vi "New Data Logging Specification (Text).vi"(5 "Decimal Places (3)":u32=3, 6 "Header Text (\"\")":string, 7 "Delimiter (Tab)":T2, 8 "error in (no error)":errorcluster, 9 "Channel Paths":T1[](array[typedef]), 10 "File Conflict Operation":T3, 11 "Base Log File Path":path) -> (0 "error out":errorcluster, 3 "Data Logging Specification Ref out":T4)   [LabVIEW 2020, in "NI_VS Data Logging API.lvlib"]
doc: "Creates a new data logging specification, which defines the channels to log and the type and base path for log files. You can log data to TDMS or text (.txt) files. You must manually select the polymorphic instance to use."
uses:
  <vilib>/NI VeriStand/Execution/DataLogging/NI_VS Data Logging API.lvlib
  <vilib>/NI VeriStand/Execution/DataLogging/DataLoggingSpecification Ref.ctl
  NationalInstruments.VeriStand.ClientAPI
  <vilib>/NI VeriStand/Execution/DataLogging/File Conflict Operation.ctl
  <vilib>/NI VeriStand/Execution/DataLogging/Delimiter.ctl
  <vilib>/NI VeriStand/Execution/DataLogging/Text Channel.ctl
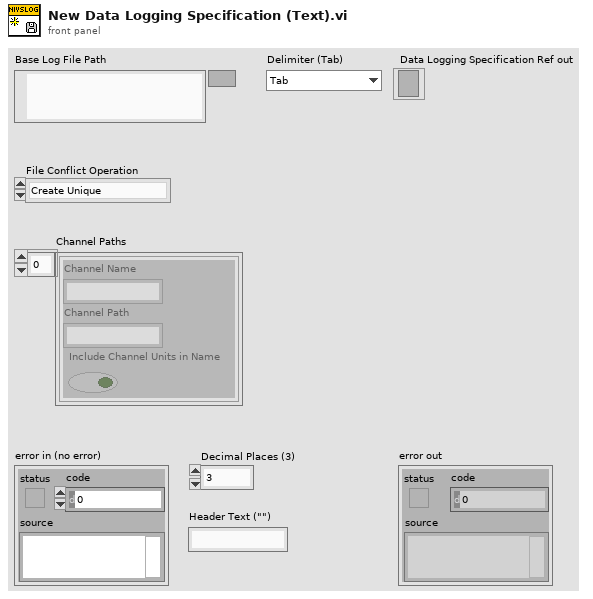
[diagram p1: front panel]
types:
  T1 = typedef "NI_VS Data Logging API.lvlib/Text Channel.ctl" = cluster{"Channel Name":string, "Channel Path":string, "Include Channel Units in Name":bool}
  T2 = typedef "NI_VS Data Logging API.lvlib/Delimiter.ctl" = enum16{"Tab", "Comma"}
  T3 = typedef "NI_VS Data Logging API.lvlib/File Conflict Operation.ctl" = enum16{"Create Unique", "Append to Existing", "Overwrite"}
  T4 = typedef "NI_VS Data Logging API.lvlib/DataLoggingSpecification Ref.ctl" = refnum<k24>
  T5 = typedef "NI_VS Data Logging API.lvlib/TextLogFile Ref.ctl" = refnum<k24>
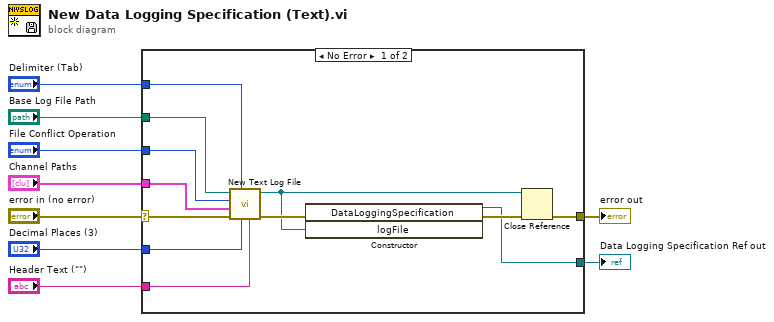
[diagram p0: block diagram]
diagram:
  n1 = case shown="No Error" "error in (no error)" {
    selector: "error in (no error)" -> [w16 w22]
    tunnel: [w18 _] -> w8
    tunnel: [w17 w22] -> w7
    tunnel: "File Conflict Operation" -> [w15 _]
    tunnel: "Base Log File Path" -> [w14 _]
    tunnel: "Delimiter (Tab)" -> [w13 _]
    tunnel: "Channel Paths" -> [w12 _]
    tunnel: "Decimal Places (3)" -> [w11 _]
    tunnel: "Header Text (\"\")" -> [w10 _]
    frame No Error {
      n2 = call <vilib>:"New Text Log File.vi"("Header Text (\"\")"=w10, "Decimal Places (3)"=w11, "Delimiter (Tab)"=w13, "error in (no error)"=w16, "Channel Paths"=w12, "File Conflict Operation"=w15, "Log File Path"=w14) -> ("error out"=w21:errorcluster, "TextLogFile Ref"=w19:T5)  [unwired: 3 in]
      n3 = constructor class="DataLoggingSpecification"(error in=w21, "logFile"=w19) -> (reference out=w18:refnum<k24>, error out=w20:errorcluster)  [unwired: 2 in, 2 out]
      n4 = Close Reference(reference=w19, error in (no error)=w20) -> (error out=w17:errorcluster)
    }
    frame Error {
    }
  }
  "error out" <- w7
  "Data Logging Specification Ref out" <- w8
